vi "Shifts gradients.vi"(1 "Activation functions, dF":dbl[][](array[numeric]) format="%.3f", 2 "Feedbacks, C":dbl[][](array[numeric]) format="%.3f", 3 "Errors":dbl[](array[numeric]) format="%.3f", 4 "Total control, U":dbl=1.0 min=1.0 max=10.0 step=1.0 format="%.3f") -> (0 "Shifts, B":dbl[](array[numeric]) format="%.3f")   [LabVIEW 2022 SP3]
uses:
  <vilib>/Analysis/baseanly.llb/Real A x B.vi
  <vilib>/Analysis/baseanly.llb/Vector x A.vi
  <vilib>/Analysis/NI_AALBase.lvlib
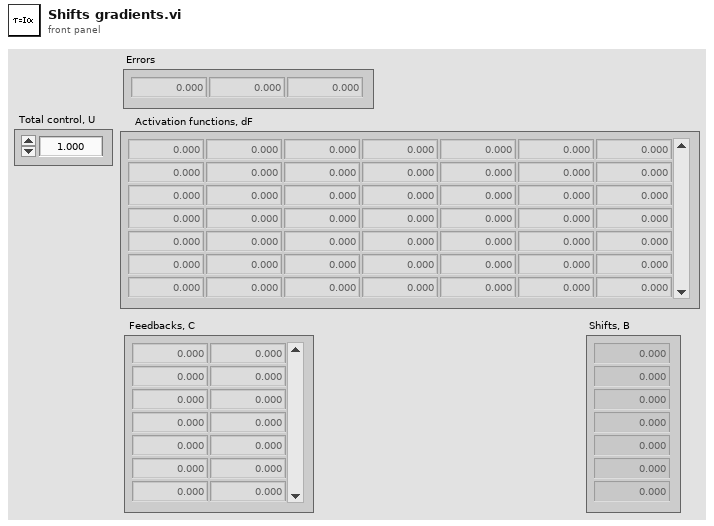
[diagram p1: front panel]
types:
  T1 = typedef "NI_Matrix.lvlib/RealMatrix.ctl" = dbl[][]
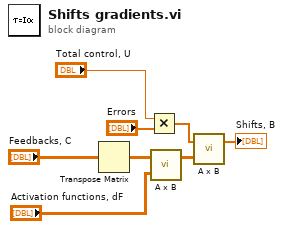
[diagram p0: block diagram]
diagram:
  n1 = Transpose Matrix(1:"Feedbacks, C") -> (0:w5:dbl[][])
  n2 = Multiply ("Multiply.vi")(x="Total control, U", y="Errors") -> (x*y=w4:dbl[])
  n3 = call-poly <vilib>:"A x B.vi"("B"="Activation functions, dF", "A"=w5) -> ("A x B"=w3:T1)  [unwired: 1 out]
  n4 = call-poly <vilib>:"A x B.vi"("Matrix A"=w3, "Vector V'"=w4) -> ("V' x A"=→"Shifts, B":dbl[])  [unwired: 1 out]
